vi "Measure Delay.vi"(0 "MSOX6004 in":refnum<class "MSOX6004.lvclass">, 1 "From Slope Edge":T2, 5 "From Channel":T3, 7 "To Channel":T3, 9 "No. Reads":i32=2000, 11 "error in (no error)":errorcluster, 12 "To Slope Edge":T2) -> (4 "MSOX6004 out":refnum<class "MSOX6004.lvclass">, 6 "Statistics":T1, 15 "error out":errorcluster)   [LabVIEW 2018, in "MSOX6004.lvlib" / "MSOX6004.lvclass"]
uses:
  MSOX6004.lvclass
  PPLs/Oscilloscope/Parent/Oscilloscope.lvlibp/Custom Controls/Analog Channels.ctl
  PPLs/Oscilloscope/Parent/Oscilloscope.lvlibp/Custom Controls/Slope Edge.ctl
  MSOX6004.lvclass/MSOX6004.ctl
  <instrlib>/Keysight InfiniiVision/Keysight InfiniiVision.lvlib
  PPLs/Oscilloscope/Parent/Oscilloscope.lvlibp
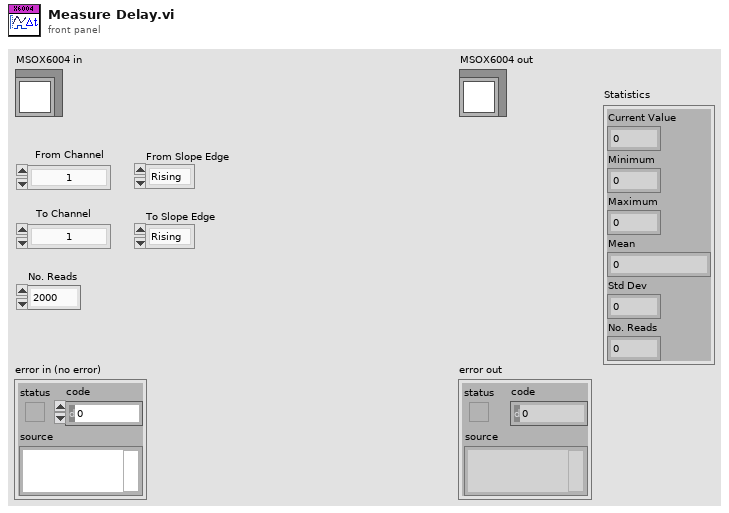
[diagram p1: front panel]
types:
  T1 = cluster{"Current Value":dbl, "Minimum":dbl, "Maximum":dbl, "Mean":dbl, "Std Dev":dbl, "No. Reads":dbl}
  T2 = typedef "Oscilloscope.lvlibp/Slope Edge.ctl" = enum16{"Rising", "Falling"}
  T3 = typedef "Oscilloscope.lvlibp/Analog Channels.ctl" = enum16{"1", "2", "3", "4", "5", "6", "7", "8", "9", "10", "11", "12", "13", "14", "15", "16"}
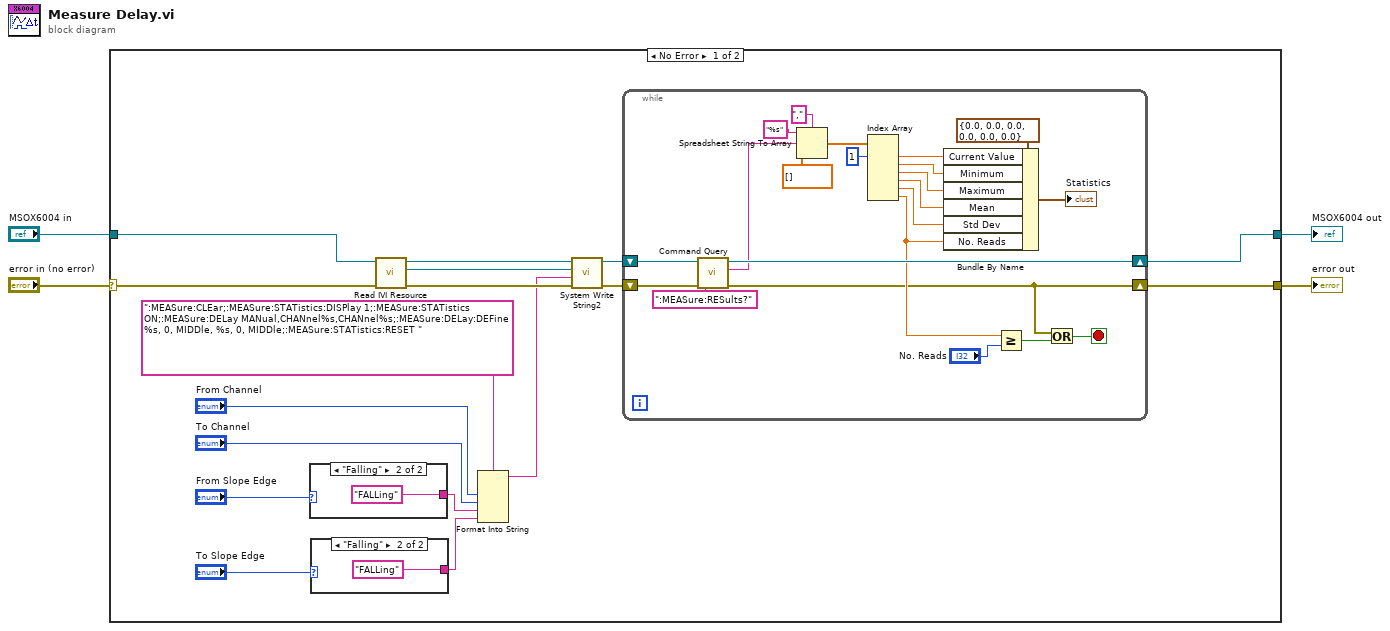
[diagram p0: block diagram]
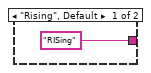
[diagram p2: hidden frame]
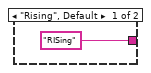
[diagram p3: hidden frame]
diagram:
  n1 = case shown="No Error" "error in (no error)" {
    selector: "error in (no error)" -> [w19 w48]
    tunnel: [w13 w48] -> w3
    tunnel: [w14 w47] -> w2
    tunnel: "MSOX6004 in" -> [w20 w47]
    frame No Error {
      n2 = case shown="\"Falling\"" "From Slope Edge" {
        tunnel: ["RISing" "FALLing"] -> w9
        frame "Rising", Default {
        }
        frame "Falling" {
        }
      }
      n3 = case shown="\"Falling\"" "To Slope Edge" {
        tunnel: ["RISing" "FALLing"] -> w10
        frame "Rising", Default {
        }
        frame "Falling" {
        }
      }
      n4 = call "Read IVI Resource.vi"("error in (no error)"=w19, "MSOX6004 in"=w20) -> ("error out"=w16:errorcluster, "IVI Resource"=w15:refnum<k15>, "MSOX6004 out"=w6:refnum<class "MSOX6004.lvclass">)  [unwired: 7 in]
      n5 = Format Into String(format string=":MEASure:CLEar;:MEASure:STATistics:DISPlay 1;:MEASure:STATistics ON;:MEASure:DELay MANual,CHANnel%s,CHANnel%s;:MEASure:DELay:DEFine %s, 0, MIDDle, %s, 0, MIDDle;:MEASure:STATistics:RESET ", "From Channel", "To Channel", w9, w10) -> (resulting string=w11:string)  [unwired: 2 in, 1 out]
      n6 = call <instrlib>:"System Write String2.vi"("error in (no error)"=w16, "Data"=w11, "instrument handle"=w15) -> ("error out"=w5:errorcluster)  [unwired: 7 in, 1 out]
      n7 = while {
        shift-right: [w44] -> w14
        shift-left: w6 -> [w46]
        shift-right: [w28] -> w13
        shift-left: w5 -> [w45]
        stop <- w27 stop-if-true
        n8 = call "Command Query.vi"("error in (no error)"=w45, "Command"=":MEASure:RESults?", "MSOX6004 in"=w46) -> ("error out"=w28:errorcluster, "Response"=w32:string, "MSOX6004 out"=w44:refnum<class "MSOX6004.lvclass">)  [unwired: 6 in]
        n9 = Spreadsheet String To Array(delimiter (Tab)=",", format string="%s", spreadsheet string=w32, array type (2D Dbl)=dbl[] []) -> (array=w40:dbl[])
        n10 = Index Array(array=w40, index #1=1 ("index")) -> (element #1=w37:dbl, element #2=w36:dbl, element #3=w35:dbl, element #4=w34:dbl, element #5=w33:dbl, element #6=w29:dbl)  [unwired: 5 in]
        n11 = Bundle By Name(cluster=T1 {"Current Value"=0.0, "Minimum"=0.0, "Maximum"=0.0, "Mean"=0.0, "Std Dev"=0.0, "No. Reads"=0.0} ("Statistics"), "Current Value"=w37, "Minimum"=w36, "Maximum"=w35, "Mean"=w34, "Std Dev"=w33, "No. Reads"=w29) -> (→"Statistics":T1)
        n12 = Greater Or Equal?(x=w29, y="No. Reads") -> (x >= y?=w25:bool)
        n13 = Or(x=w28, y=w25) -> (x .or. y?=w27:bool)
      }
    }
    frame Error {
    }
  }
  "error out" <- w3
  "MSOX6004 out" <- w2
